vi "test write header.vi"() -> ()   [LabVIEW 2014]
uses:
  XDisplay/POLARIS IMAQ Display.xctl
  POLARIS Vision utility.lvlib
panel:
  out "error out":errorcluster
  out "Actual Index":i32
  out "Image":T1(plugin-control)
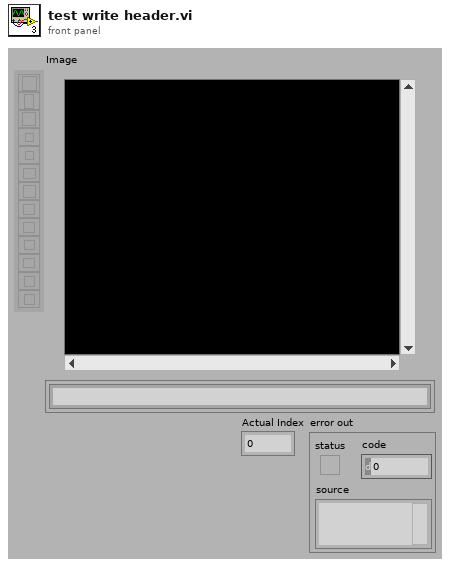
[diagram p1: front panel]
types:
  T1 = typedef "IMAQ Image.ctl" = refnum<image>
  T2 = typedef "Image Type" = u32
  T3 = cluster{"Global Rectangle":i32[], "Contours":cluster{"Contour Type":u32, "ROI Type":u32, "Points":i32[]}[]}
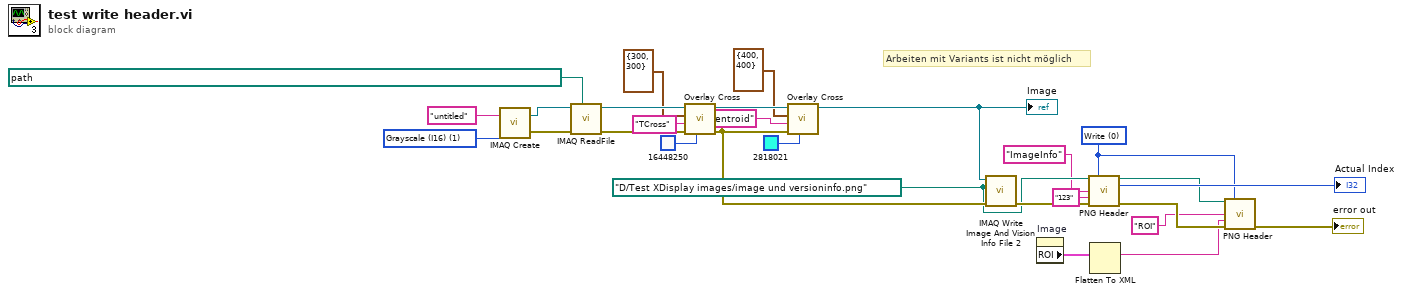
[diagram p0: block diagram]
diagram:
  w5 = u16 0 items=["Write", "read"] ("Mode")
  w11 = path "D:/Test XDisplay images/image und versioninfo.png" ("File Path")
  w27 = T2 1 items=["Grayscale (U8)", "Grayscale (I16)", "Grayscale (SGL)", "Complex (CSG)", "RGB (U32)", "HSL (U32)", "RGB (U64)", "Grayscale (U16)"] ("Image Type")
  # "Arbeiten mit Variants ist nicht möglich"
  n1 = call "IMAQ Create"("Image Name"="untitled", "Image Type"=w27) -> ("New Image"=w26:T1, "error out"=w25:errorcluster)  [unwired: 3 in]
  n2 = call "IMAQ ReadFile"("File Path"=path "C:/Users/user/Desktop/Foki/1408 - 05 - neue Düse/A2 - 2014-08-05, 10.34.27, q=0,36, A=546,2µm2.png", "error in (no error)"=w25, "Image"=w26) -> ("error out"=w23:errorcluster, "Image Out"=w24:T1)  [unwired: 4 in, 3 out]
  n3 = call "Overlay Cross.vi"("Color"=u32 16448250, "error in (no error)"=w23, "Overlay Group"="TCross", "point"=cluster{"x":i16, "y":i16} {"x"=300, "y"=300}, "Image In"=w24) -> ("error out"=w19:errorcluster, "Image Out"=w18:T1)  [unwired: 4 in]
  n4 = call "Overlay Cross.vi"("Color"=u32 2818021, "error in (no error)"=w19, "Overlay Group"="Centroid", "point"=cluster{"x":i16, "y":i16} {"x"=400, "y"=400}, "Image In"=w18) -> ("Image Out"=w17:T1)  [unwired: 4 in, 1 out]
  "Image" <- w17
  n5 = call "IMAQ Write Image And Vision Info File 2"("error in (no error)"=w19, "File Path"=w11, "Image"=w17) -> ("error out"=w12:errorcluster)  [unwired: 7 in, 1 out]
  n6 = property on="Image" class="ImageControl"() -> ("ROI"=w2:T3)  [unwired: 2 in, 2 out]
  n7 = call "PNG Header.vi"("Path In"=w11, "Mode"=w5, "header in"="ImageInfo", "string in"="123", "error in (no error)"=w12) -> ("pathOut"=w4:path, "Actual Index"=→"Actual Index":i32, "error out"=w7:errorcluster)  [unwired: 6 in, 2 out]
  n8 = Flatten To XML(anything=w2) -> (xml string=w1:string)
  n9 = call "PNG Header.vi"("Path In"=w4, "Mode"=w5, "header in"="ROI", "string in"=w1, "error in (no error)"=w7) -> ("error out"=→"error out":errorcluster)  [unwired: 6 in, 4 out]
